vi "ep_Public Event Inf to String.vi"(8 "error in":errorcluster, 10 "initial string":string, 11 "task in":T1={"file refnums"=[], "Data Object"=refnum, "config info"={"station_name"="", "rec_dev_id"="", "rev_year"=1999.0, "TT"=0, "##A"=0, "##D"=0, "analog channel info"=[], "status channel info"=[], "lf"=-inf, "nrates"=65535, "samp info"=[], "initial timestamp"=timestamp(0 s since 1904-01-01), "trigger timestamp"=timestamp(0 s since 1904-01-01), "ft"=enum."Binary", "timemult"=1.0}, "public inf content"={"Source"="", "Record Type"=enum."Fault", "Phase ID"="", "Event Description"="", "Device ID"="", "Distance of Fault"=-1.0, "Distance Unit"=enum."Miles", "Max_Current"=inf, "Min_Current"=-inf, "Max_Voltage"=inf, "Min_Voltage"=-inf, "EventNoteCount"=0, "Event Information"=[]}, "private inf content"=[], "internal buffers"={"start index"=1, "config to public inf"=enum."disabled", "static config info"="", "static file_des record inf"="", "static file_des channel inf"="", "public inf"="", "private inf"=""}} {"public inf content"."Event Information"."min sample number" max=9999999999; "public inf content"."Event Information"."max sample number" max=9999999999; "config info"."nrates" max=999; "config info"."status channel info"."Dn" min=1 max=999999; "config info"."analog channel info"."An" min=1 max=999999; "config info"."trigger timestamp" format="%<%H:%M:%S%6u\n%d/%m/%Y>T"; "config info"."initial timestamp" format="%<%H:%M:%S%6u\n%d/%m/%Y>T"; "config info"."##D" max=999999; "config info"."##A" max=999999; "config info"."TT" min=1 max=999999; "config info"."rev_year" min=1999.0 max=1999.0}) -> (0 "error out":errorcluster, 2 "public event inf appended":string, 3 "dup task":T1={"file refnums"=[], "Data Object"=refnum, "config info"={"station_name"="", "rec_dev_id"="", "rev_year"=1999.0, "TT"=0, "##A"=0, "##D"=0, "analog channel info"=[], "status channel info"=[], "lf"=-inf, "nrates"=65535, "samp info"=[], "initial timestamp"=timestamp(0 s since 1904-01-01), "trigger timestamp"=timestamp(0 s since 1904-01-01), "ft"=enum."Binary", "timemult"=1.0}, "public inf content"={"Source"="", "Record Type"=enum."Fault", "Phase ID"="", "Event Description"="", "Device ID"="", "Distance of Fault"=-1.0, "Distance Unit"=enum."Miles", "Max_Current"=inf, "Min_Current"=-inf, "Max_Voltage"=inf, "Min_Voltage"=-inf, "EventNoteCount"=0, "Event Information"=[]}, "private inf content"=[], "internal buffers"={"start index"=1, "config to public inf"=enum."disabled", "static config info"="", "static file_des record inf"="", "static file_des channel inf"="", "public inf"="", "private inf"=""}} {"public inf content"."Event Information"."min sample number" max=9999999999; "public inf content"."Event Information"."max sample number" max=9999999999; "config info"."nrates" max=999; "config info"."status channel info"."Dn" min=1 max=999999; "config info"."analog channel info"."An" min=1 max=999999; "config info"."trigger timestamp" format="%<%H:%M:%S%6u\n%d/%m/%Y>T"; "config info"."initial timestamp" format="%<%H:%M:%S%6u\n%d/%m/%Y>T"; "config info"."##D" max=999999; "config info"."##A" max=999999; "config info"."TT" min=1 max=999999; "config info"."rev_year" min=1999.0 max=1999.0})   [LabVIEW 2014, in "NI_EP_COMTRADE.lvlib"]
uses:
  <vilib>/addons/Electrical Power/File IO/NI_EP_COMTRADE.lvlib
  <vilib>/addons/Electrical Power/File IO/COMTRADE/typedefs/ep_Task.ctl
  <vilib>/addons/Electrical Power/File IO/COMTRADE/typedefs/ep_Config Info.ctl
  <vilib>/addons/Electrical Power/File IO/COMTRADE/typedefs/ep_Analog Channel Info.ctl
  <vilib>/addons/Electrical Power/File IO/COMTRADE/typedefs/ep_Status Channel Info.ctl
  <vilib>/addons/Electrical Power/File IO/COMTRADE/typedefs/ep_File Format.ctl
  <vilib>/addons/Electrical Power/File IO/COMTRADE/typedefs/ep_Public Inf Content.ctl
  <vilib>/addons/Electrical Power/File IO/COMTRADE/typedefs/ep_Public Event Inf.ctl
  <vilib>/addons/Electrical Power/File IO/COMTRADE/typedefs/ep_Private Inf Content.ctl
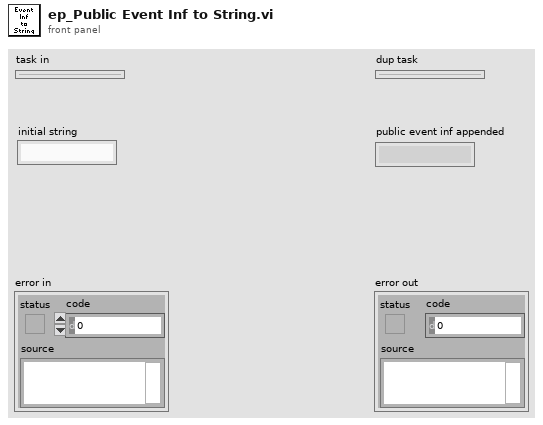
[diagram p1: front panel]
types:
  T1 = typedef "NI_EP_COMTRADE.lvlib/ep_Task.ctl" = cluster{"file refnums":refnum<file>[], "Data Object":refnum<k20>, "config info":T2, "public inf content":T6, "private inf content":T8, "internal buffers":cluster{"start index":u32, "config to public inf":enum16{"disabled", "enabled", "buffered"}, "static config info":string, "static file_des record inf":string, "static file_des channel inf":string, "public inf":string, "private inf":string}}
  T2 = typedef "NI_EP_COMTRADE.lvlib/ep_Config Info.ctl" = cluster{"station_name":string, "rec_dev_id":string, "rev_year":dbl, "TT":u32, "##A":u32, "##D":u32, "analog channel info":T3[], "status channel info":T4[], "lf":sgl, "nrates":u16, "samp info":cluster{"samp":sgl, "endsamp":u32}[], "initial timestamp":timestamp, "trigger timestamp":timestamp, "ft":T5, "timemult":sgl}
  T3 = typedef "NI_EP_COMTRADE.lvlib/ep_Analog Channel Info.ctl" = cluster{"An":u32, "ch_id":string, "ph":string, "ccbm":string, "uu":string, "a":sgl, "b":sgl, "skew":sgl, "min":i32, "max":i32, "primary":sgl, "secondary":sgl, "PS":enum16{"P", "S"}}
  T4 = typedef "NI_EP_COMTRADE.lvlib/ep_Status Channel Info.ctl" = cluster{"Dn":u32, "ch_id":string, "ph":string, "ccbm":string, "Y":bool}
  T5 = typedef "NI_EP_COMTRADE.lvlib/ep_File Format.ctl" = enum16{"ASCII", "Binary"}
  T6 = typedef "NI_EP_COMTRADE.lvlib/ep_Public Inf Content.ctl" = cluster{"Source":string, "Record Type":enum16{"Fault", "Unknown", "Misoperation", "Close", "Trip", "Reclose", "Power swing", "Simulation"}, "Phase ID":string, "Event Description":string, "Device ID":string, "Distance of Fault":dbl, "Distance Unit":enum16{"Miles", "Kilometers", "Percent of line", "Percent of setting", "Ohms"}, "Max_Current":dbl, "Min_Current":dbl, "Max_Voltage":dbl, "Min_Voltage":dbl, "EventNoteCount":u32, "Event Information":T7[]}
  T7 = typedef "NI_EP_COMTRADE.lvlib/ep_Public Event Inf.ctl" = cluster{"channel number":u32, "max value":dbl, "min value":dbl, "max sample number":u64, "min sample number":u64, "max sample text":string[], "min sample text":string[]}
  T8 = typedef "NI_EP_COMTRADE.lvlib/ep_Private Inf Content.ctl" = cluster{"Section Header":string, "Entry Names":string[], "Entry Values":string[]}[]
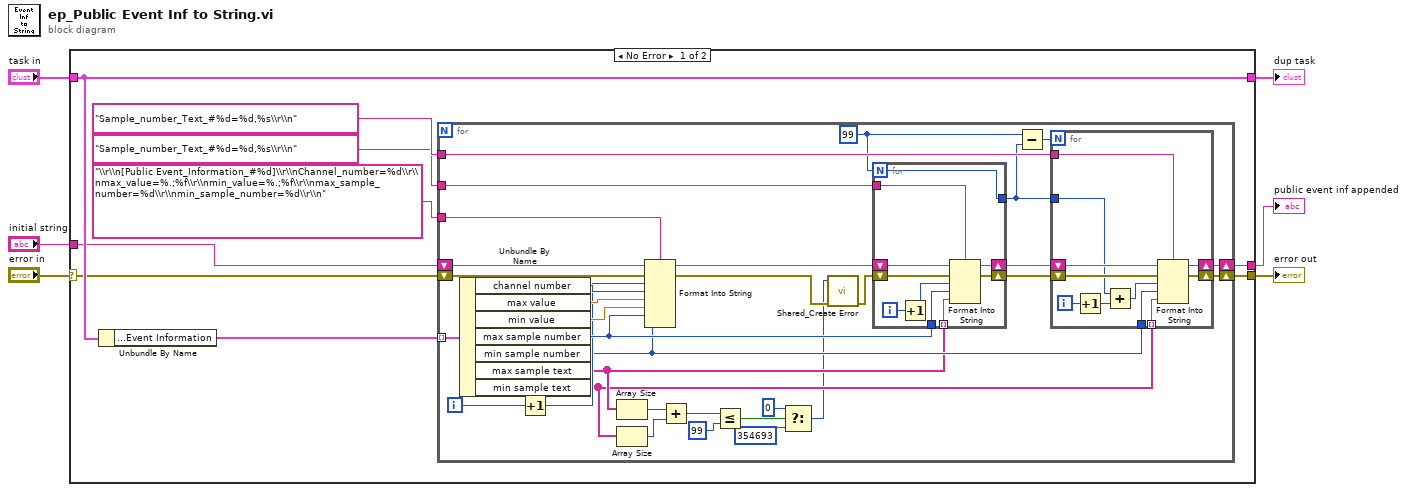
[diagram p0: block diagram]
diagram:
  n1 = case shown="No Error" "error in" {
    selector: "error in" -> [w13 w70]
    tunnel: "task in" -> [w15 w71]
    tunnel: [w15 w71] -> w4
    tunnel: [w11 w70] -> w3
    tunnel: [w12 _] -> w2
    tunnel: "initial string" -> [w10 _]
    frame No Error {
      n2 = Unbundle By Name(w15) -> ("public inf content.Event Information"=w14:T7[])
      n3 = for {
        tunnel: w14 -> [w48] mode=indexing
        shift-right: [w34] -> w11
        shift-left: w13 -> [w45]
        shift-right: [w35] -> w12
        shift-left: w10 -> [w44]
        tunnel: "\\r\\n[Public Event_Information_#%d]\\r\\nChannel_number=%d\\r\\nmax_value=%.;%f\\r\\nmin_value=%.;%f\\r\\nmax_sample_number=%d\\r\\nmin_sample_number=%d\\r\\n" ("format string") -> [w33]
        tunnel: "Sample_number_Text_#%d=%d,%s\\r\\n" ("format string") -> [w32]
        tunnel: "Sample_number_Text_#%d=%d,%s\\r\\n" ("format string") -> [w31]
        i -> [w37]
        w16 = 99
        n4 = Unbundle By Name(w48) -> ("channel number"=w43:u32, "max value"=w47:dbl, "min value"=w46:dbl, "max sample number"=w41:u64, "min sample number"=w36:u64, "max sample text"=w28:string[], "min sample text"=w27:string[])
        n5 = Increment(x=w37) -> (x+1=w38:i32)
        n6 = Array Size(array=w28) -> (size(s)=w30:i32)
        n7 = Array Size(array=w27) -> (size(s)=w29:i32)
        n8 = Format Into String(format string=w33, initial string=w44, error in=w45, w38, w43, w47, w46, w41, w36) -> (resulting string=w42:string, error out=w24:errorcluster)
        n9 = Add(x=w30, y=w29) -> (x+y=w21:i32)
        n10 = Less Or Equal?(x=w21, y=99) -> (x <= y?=w20:bool)
        n11 = Select(t=0 ("code"), s=w20, f=354693) -> (s? t:f=w22:i32)
        n12 = call <vilib>:"Shared_Create Error.vi"("error in (no error)"=w24, "error code (0)"=w22) -> ("error out"=w23:errorcluster)  [unwired: 9 in]
        n13 = for {
          N: w16 -> [w61]
          shift-right: [w68] -> w40
          shift-left: w23 -> [w69]
          tunnel: w28 -> [w67] mode=indexing
          shift-right: [w65] -> w39
          shift-left: w42 -> [w66]
          tunnel: w41 -> [w64]
          tunnel: [w61] -> w17
          tunnel: w31 -> [w60]
          i -> [w62]
          n14 = Increment(x=w62) -> (x+1=w63:i32)
          n15 = Format Into String(format string=w60, initial string=w66, error in=w69, w63, w64, w67) -> (resulting string=w65:string, error out=w68:errorcluster)
        }
        n16 = Subtract(x=w16, y=w17) -> (x-y=w18:i32)
        n17 = for {
          N: w18 -> [_]
          shift-right: [w58] -> w34
          shift-left: w40 -> [w59]
          tunnel: w27 -> [w57] mode=indexing
          shift-right: [w55] -> w35
          shift-left: w39 -> [w56]
          tunnel: w36 -> [w54]
          tunnel: w17 -> [w50]
          tunnel: w32 -> [w49]
          i -> [w53]
          n18 = Increment(x=w53) -> (x+1=w52:i32)
          n19 = Add(x=w50, y=w52) -> (x+y=w51:i32)
          n20 = Format Into String(format string=w49, initial string=w56, error in=w59, w51, w54, w57) -> (resulting string=w55:string, error out=w58:errorcluster)
        }
      }
    }
    frame Error {
    }
  }
  "public event inf appended" <- w2
  "dup task" <- w4
  "error out" <- w3
